vi "test.vi"() -> ()   [LabVIEW 2013]
uses:
  TypeDef/FrontPanelKEITHLEY2182_KEITHLEY6221.ctl
  Keithley 622x lib/Configure/2182 -A/Low Lewel/Typedefs/KE2182 -- Params.ctl
  Keithley 622x lib/Configure/Source/Typedefs/KE622x -- Current Range.ctl
  Keithley 622x lib/Configure/Source/Typedefs/KE622x -- Current Level.ctl
  Keithley 622x lib/Configure/Source/Typedefs/KE622x -- Voltage Limit.ctl
  Keithley 622x lib/Configure/Output/Typedefs/KE6221 -- Output Response.ctl
  graph/DysplayGraph.ctl
  Keithley 622x lib/Keithly user program.lvlib
panel:
  out "Output Values of Device":T1 {"KEITHLEY 2182 & KEITHLEY 6221" format="%#_6e"}
  in  "DisplayGraphsTable":T3 {"KEITHLEY2182andKEITHLEY6221"."Y is" items=["Time", "Volt", "Current", "Resist"]; "KEITHLEY2182andKEITHLEY6221"."X is" items=["Time", "Volt", "Current", "Resist"]}
  in  "Other Devices":cluster{"Boolean":bool}
  in  "KEITHLEY 2182 & KEITHLEY 6221":T4={"KEITHLEY ON/OFF"=FALSE, "VISA KEITHLEY resource name"="GPIB0::12::INSTR", "2182 -A Params"={"Auto Range?"=FALSE, "Man / Selected\n       Range"=enum."10mV", "Enable Digital\n       Filter?"=FALSE, "Filter Type"=enum."Movin", "Filter Count"=1, "      Filter\nWindow (%)"=0.01, "Enable Analog\n       Filter?"=FALSE, "NPLCs"=5}, "KEITHLEY CURRENT ON/OFF"=FALSE, "6221 Params"={"Current Range"={"Auto Range?"=FALSE, "Man / Selected\n        Range"=enum."2nA"}, "Current Level (A)"=0.1, "Voltage Limit (V)"=10.0, "KE6221 Output Response"=enum."Fast", "Analog Filter State"=enum."Off"}, "Step Mode\nParams"=FALSE, "Step Mode"={"Front Point (A)"=0.1, "Start Point (A)"=0.1, "Back Point (A)"=0.1, "Step(A)"=0.1, "Time step (ms)"=0.0, "N cycle"=0, "Sweeping"=enum."Off Sweeping", "Go to"=enum."Star Point"}} {"Step Mode"."N cycle" min=1 step=1; "Step Mode"."Time step (ms)" min=0.0 step=1.0; "Step Mode"."Step(A)" min=-0.105 max=0.105 format="%.4p"; "Step Mode"."Back Point (A)" min=-0.105 max=0.105 format="%.4p"; "Step Mode"."Start Point (A)" min=-0.105 max=0.105 format="%.4p"; "Step Mode"."Front Point (A)" min=-0.105 max=0.105 format="%.4p"; "6221 Params"."Current Level (A)" min=-0.105 max=0.105 format="%.4p"; "6221 Params"."Voltage Limit (V)" min=0.1 max=105.0 step=0.01 format="%.2p"; "2182 -A Params"."NPLCs" min=1 max=10; "2182 -A Params"."Filter\nWindow (%)" min=0.01 max=10.0 step=0.01 format="%.2f"; "2182 -A Params"."Filter Count" min=1 max=100}
  in  "Main menu":T10
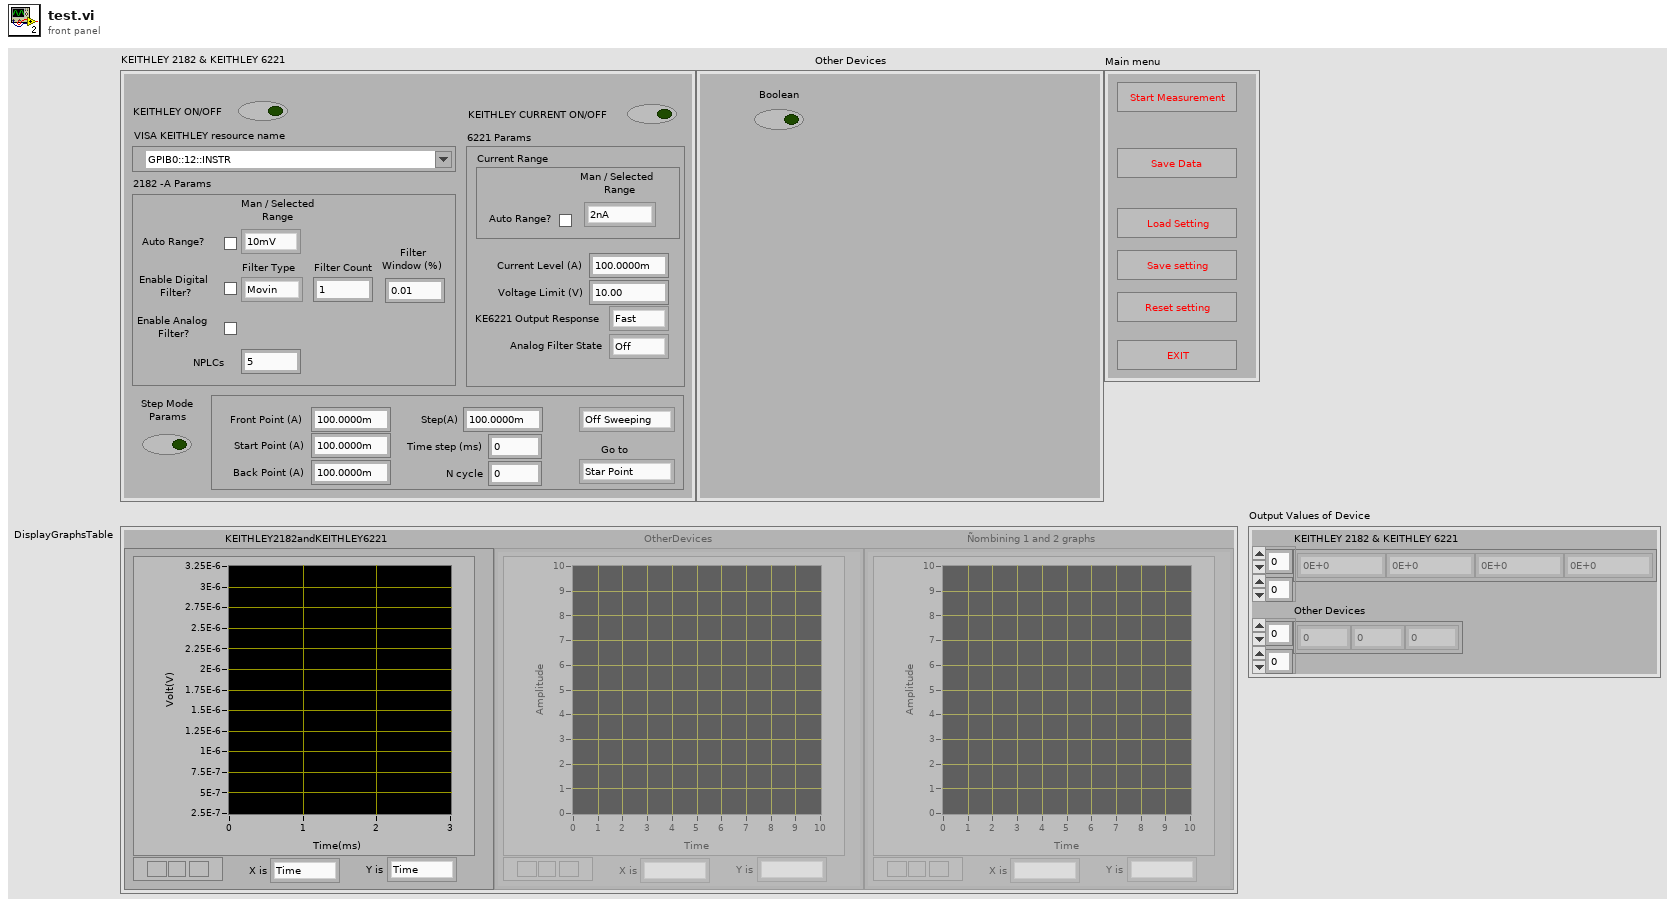
[diagram p1: front panel]
types:
  T1 = cluster{"KEITHLEY 2182 & KEITHLEY 6221":dbl[][], "Other Devices":dbl[][]}
  T2 = typedef "DysplayGraph.ctl" = cluster{"Graph":cluster{"X":dbl, "Y":dbl}[], "X is":u16, "Y is":u16}
  T3 = cluster{"KEITHLEY2182andKEITHLEY6221":T2, "OtherDevices":T2, "Ñombining 1 and 2 graphs ":T2}
  T4 = typedef "FrontPanelKEITHLEY2182_KEITHLEY6221.ctl" = cluster{"KEITHLEY ON/OFF":bool, "VISA KEITHLEY resource name":refnum<visa-resource-name>, "2182 -A Params":T5, "KEITHLEY CURRENT ON/OFF":bool, "6221 Params":cluster{"Current Range":T6, "Current Level (A)":T7, "Voltage Limit (V)":T8, "KE6221 Output Response":T9, "Analog Filter State":enum16{"Off", "On"}}, "Step Mode\nParams":bool, "Step Mode":cluster{"Front Point (A)":T7, "Start Point (A)":T7, "Back Point (A)":T7, "Step(A)":T7, "Time step (ms)":dbl, "N cycle":i32, "Sweeping":enum16{"Off Sweeping", "On Sweeping"}, "Go to":enum16{"Star Point", "Back Point"}}}
  T5 = typedef "Keithly user program.lvlib/KE2182 -- Params.ctl" = cluster{"Auto Range?":bool, "Man / Selected\n       Range":enum16{"10mV", "100mV", "1V", "10V", "100V"}, "Enable Digital\n       Filter?":bool, "Filter Type":enum16{"Movin", "Repeat"}, "Filter Count":u32, "      Filter\nWindow (%)":dbl, "Enable Analog\n       Filter?":bool, "NPLCs":u32}
  T6 = typedef "Keithly user program.lvlib/KE622x -- Current Range.ctl" = cluster{"Auto Range?":bool, "Man / Selected\n        Range":enum16{"2nA", "20nA", "200nA", "2uA", "20uA", "200uA", "2mA", "20mA", "100mA"}}
  T7 = typedef "Keithly user program.lvlib/KE622x -- Current Level.ctl" = dbl
  T8 = typedef "Keithly user program.lvlib/KE622x -- Voltage Limit.ctl" = dbl
  T9 = typedef "Keithly user program.lvlib/KE6221 -- Output Response.ctl" = enum16{"Fast", "Slow"}
  T10 = cluster{"Measurement":bool, "Save Data":bool, "LoadSetting":bool, "Save setting":bool, "Reset setting":bool, "Exit":bool}
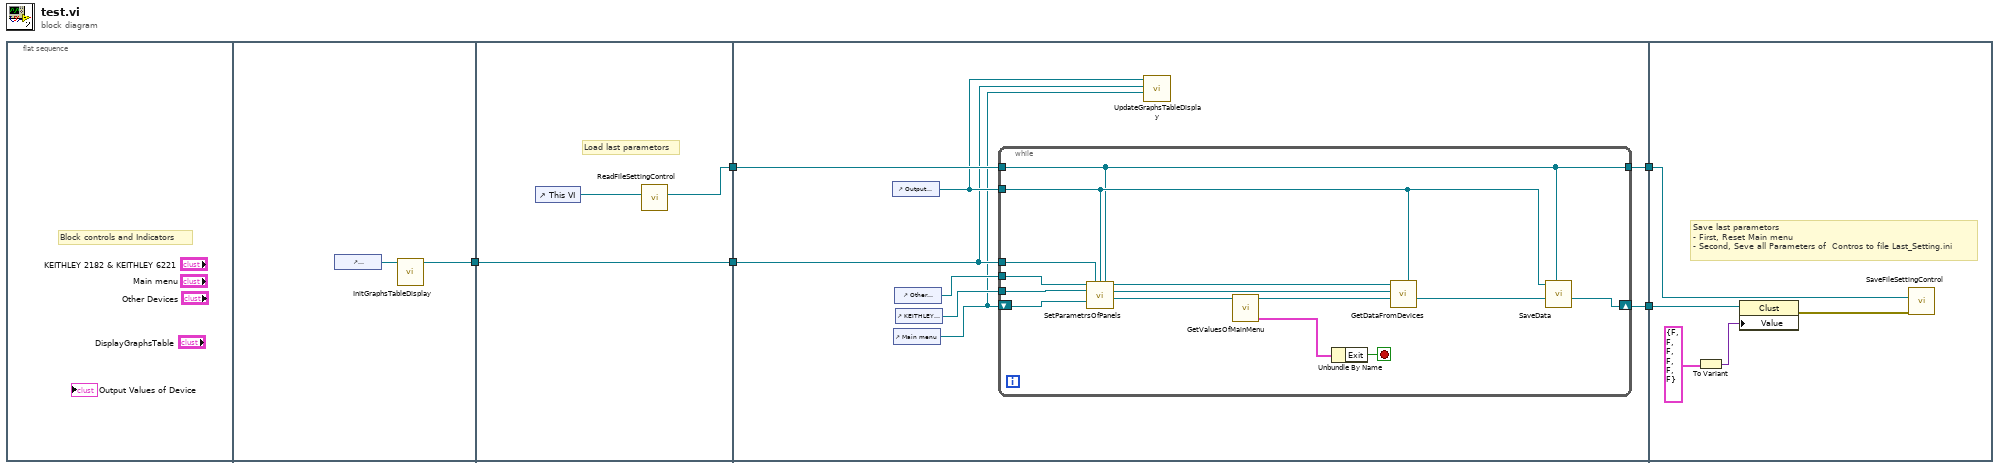
[diagram p0: block diagram]
diagram:
  n1 = flat-sequence {
    tunnel: [w6] -> w1
    tunnel: [w9] -> w4
    tunnel: [w8] -> w2
    tunnel: w1 -> [w8]
    tunnel: [w18] -> w5
    tunnel: w4 -> [w17]
    tunnel: [w16] -> w3
    tunnel: w2 -> [w12]
    tunnel: w5 -> [w35]
    tunnel: w3 -> [w33]
    frame #0 {
      # "Block controls and Indicators"
    }
    frame #1 {
      n2 = control-ref of="DisplayGraphsTable"() -> (w7:refnum<vi>)
      n3 = call "InitGraphsTableDisplay.vi"("DisplayGraphsTable_In"=w7) -> ("DisplayGraphsTable_Out"=w6:refnum<vi>)  [unwired: 10 in]
    }
    frame #2 {
      # "Load last parametors"
      n4 = control-ref of="This VI"() -> (w10:refnum<vi>)
      n5 = call "ReadFileSettingControl.vi"("ThisVI_In"=w10) -> ("ThisVI_Out"=w9:refnum<vi>)  [unwired: 10 in]
    }
    frame #3 {
      n6 = control-ref of="Output Values of Device"() -> (w13:refnum<vi>)
      n7 = control-ref of="Main menu"() -> (w11:refnum<vi>)
      n8 = control-ref of="Other Devices"() -> (w15:refnum<vi>)
      n9 = control-ref of="KEITHLEY 2182 & KEITHLEY 6221"() -> (w14:refnum<vi>)
      n10 = while {
        tunnel: w17 -> [w19]
        tunnel: [w19] -> w16
        shift-right: [w28] -> w18
        shift-left: w11 -> [w21]
        tunnel: w12 -> [w23]
        tunnel: w15 -> [w25]
        tunnel: w14 -> [w24]
        tunnel: w13 -> [w20]
        stop <- w32 stop-if-true
        n11 = call "SetParametrsOfPanels.vi"("OtherDivice_In"=w25, "DisplayGraphsTable_In"=w23, "OutputValuesOfDevices"=w20, "This VI"=w19, "KEITHLEY 2182 & KEITHLEY 6221_In"=w24, "MainMenu_In"=w21) -> ("Cluster out"=w27:refnum<vi>, "KEITHLEY 2182 & KEITHLEY 6221_Out"=w31:refnum<vi>, "Main menu out"=w22:refnum<vi>)  [unwired: 7 in]
        n12 = call "GetValuesOfMainMenu.vi"("MainMenu_In"=w22) -> ("ValuesOfMainMenu"=w26:T10, "MainMenu_Out"=w30:refnum<vi>)  [unwired: 9 in]
        n13 = Unbundle By Name(w26) -> ("Exit"=w32:bool)
        n14 = call "GetDataFromDevices.vi"("Output Values of Device"=w20, "Main menu in"=w30, "KEITHLEY 2182 & KEITHLEY 6221_In"=w31, "Cluster in"=w27) -> ("Main menu out"=w29:refnum<vi>)  [unwired: 5 in, 2 out]
        n15 = call "SaveData.vi"("ThisVI_In"=w19, "Main menu in"=w29, "Output Values of Device"=w20) -> ("Main menu out"=w28:refnum<vi>)  [unwired: 8 in]
      }
      n16 = call "UpdateGraphsTableDisplay.vi"("MainMenu_In"=w11, "DisplayGraphsTable_In"=w12, "Output Values of Device"=w13) -> ()  [unwired: 9 in]
    }
    frame #4 {
      # "Save last parametors\n- First, Reset Main menu\n- Second, Seve all Parameters of  Contros to file Last_Setting.ini"
      n17 = To Variant(anything=T10 {"Measurement"=FALSE, "Save Data"=FALSE, "LoadSetting"=FALSE, "Save setting"=FALSE, "Reset setting"=FALSE, "Exit"=FALSE} ("Main menu")) -> (Variant=w37:variant)
      n18 = property class="Clust"(reference=w35, "Value"=w37) -> (error out=w34:errorcluster)  [unwired: 1 in, 1 out]
      n19 = call "SaveFileSettingControl.vi"("error in"=w34, "This VI"=w33) -> ()  [unwired: 9 in, 1 out]
    }
  }
